vi "Fetch (Waveform To File).vi"(7 "Filename (C:\\data.txt)":path=path "C:/data.txt", 8 "error in (no error)":errorcluster, 9 "Maximum Time (200000ms)":u32=200000, 10 "Channel (0:Channel1)":u16(ring) items=["Channel1", "Channel2", "Channel3", "Channel4", "Math1", "Math2", "Math3", "Math3", "Reference1", "Reference2", "Reference3", "Reference4"], 11 "VISA resource name":refnum<visa-resource-name>) -> (0 "error out":errorcluster, 3 "VISA resource name out":refnum<visa-resource-name>)   [LabVIEW 2011, in "Tektronix 7000 Series.lvlib"]
doc: "Returns to a file the waveform that an oscilloscope acquires for a channel you specify. An acquisition that you initiate before calling this VI generates the waveform.\n\nYou first enable channels with the Configure Channel VI. Then you use the Initiate VI to start an acquisition on the enabled channels. An oscilloscope concurrently acquires waveforms for these channels and returns them in a file.\n\n<B>Note</B>: Use the Fetch Waveform To File VI only with other low-level VIs, such as the Initiate VI, the Abort VI, and the Fetch Waveform VI."
uses:
  Tektronix 7000 Series.lvlib
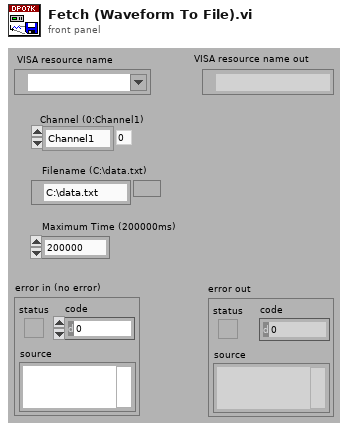
[diagram p1: front panel]
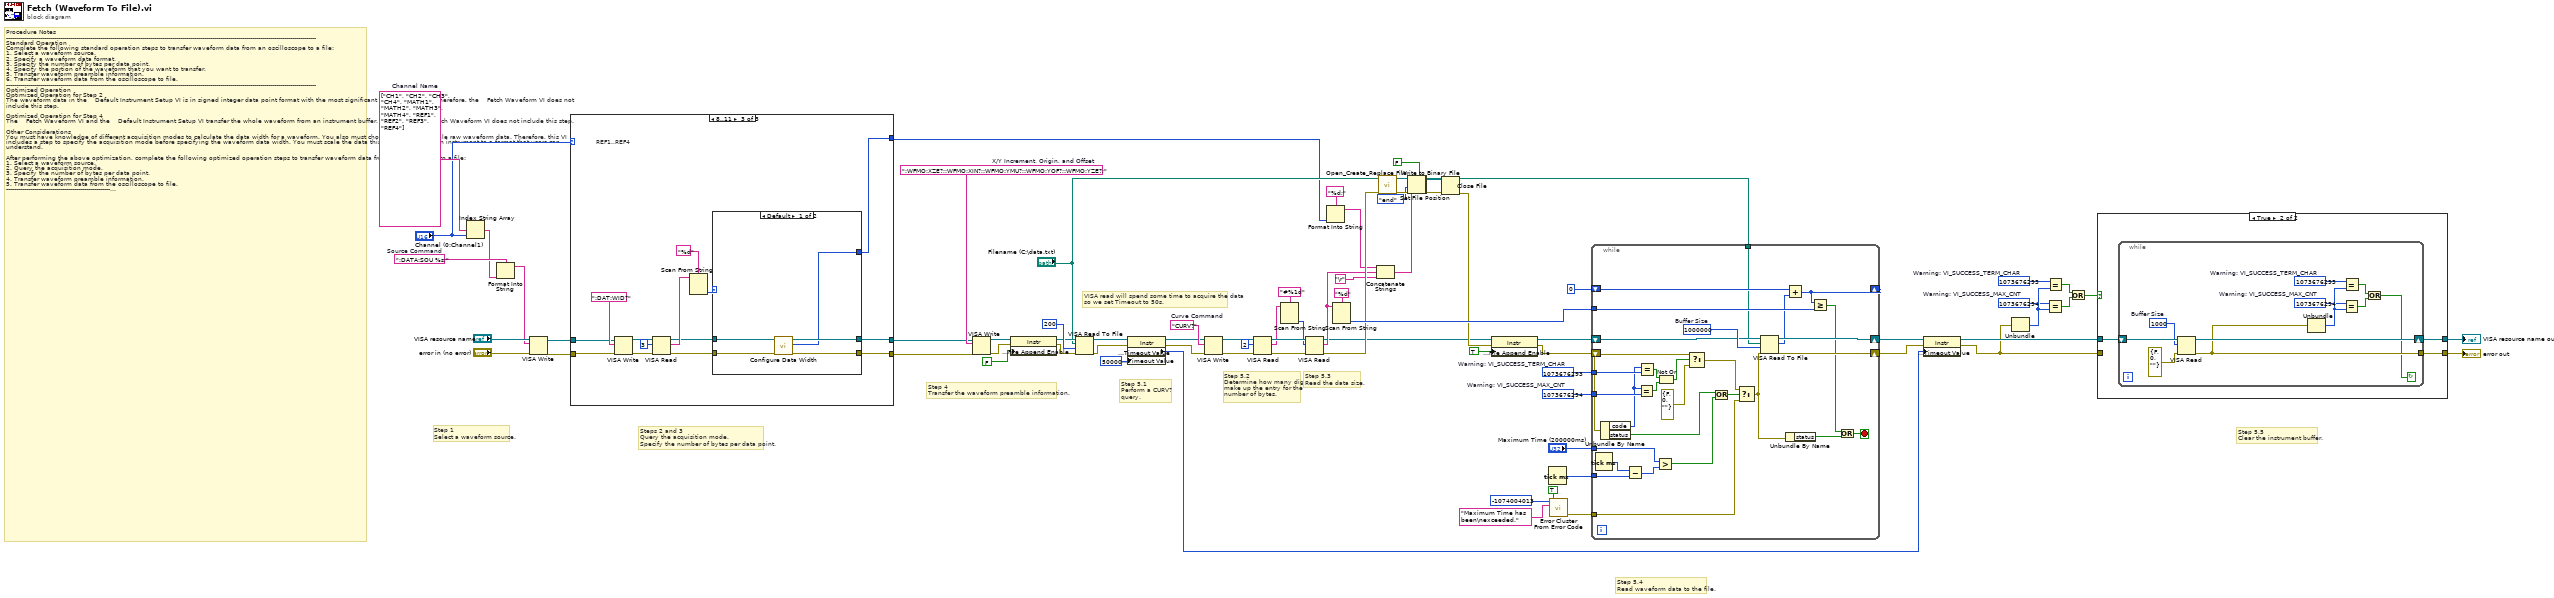
[diagram p0: block diagram]
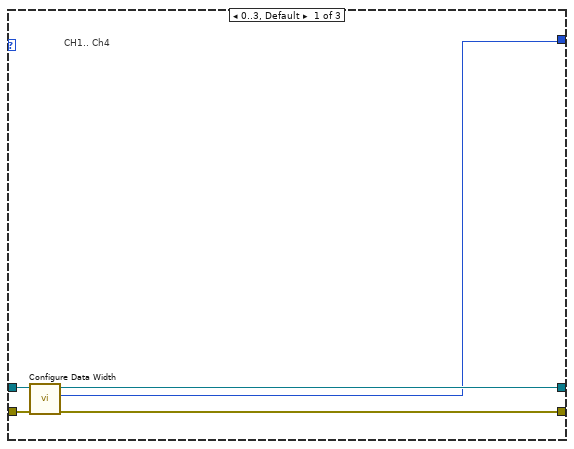
[diagram p2: hidden frame]
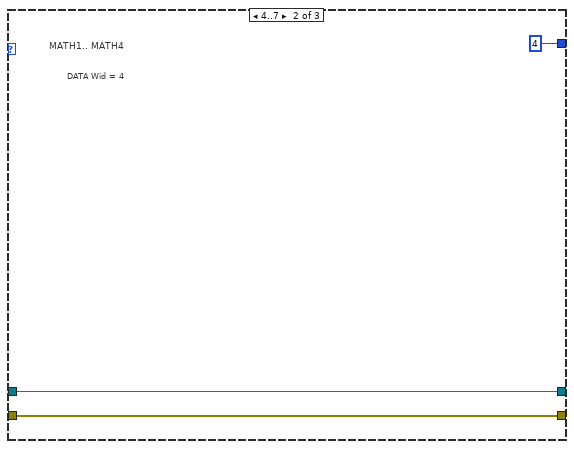
[diagram p3: hidden frame]
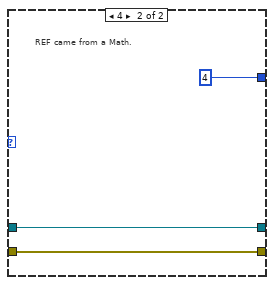
[diagram p4: hidden frame]
diagram:
  w51 = string[] ["CH1", "CH2", "CH3", "CH4", "MATH1", "MATH2", "MATH3", "MATH4", "REF1", "REF2", "REF3", "REF4"]  # Channel Name
  w57 = 1073676294  # Warning: VI_SUCCESS_MAX_CNT
  w58 = 1073676293  # Warning: VI_SUCCESS_TERM_CHAR
  w61 = 1073676294  # Warning: VI_SUCCESS_MAX_CNT
  w60 = 1073676293  # Warning: VI_SUCCESS_TERM_CHAR
  w75 = "CURV?"  # Curve Command
  w77 = ":DATA:SOU %s;"  # Source Command
  w46 = ":WFMO:XZE?;:WFMO:XIN?;:WFMO:YMU?;:WFMO:YOF?;:WFMO:YZE?;"  # X/Y Increment, Origin, and Offset
  # "VISA read will spend some time to acquire the data \nso we set Timeout to 50s."
  # "Step 4\nTransfer the waveform preamble information."
  # "Step 1\nSelect a waveform source."
  # "Steps 2 and 3\nQuery the acquisition mode. \nSpecify the number of bytes per data point."
  # "Procedure Notes\n-----------------------------------------------------------------------------------------------------------------------------------------------------------\nStandard Operation\nComplete the following standard operation steps to transfer waveform data from an oscilloscope to a file:\n1. Select a waveform source.\n2. Specify a waveform data format.\n3. Specify the number of bytes per data point.\n4. Specify the portion of the waveform that you want to transfer.\n5. Transfer waveform preamble information.\n6. Transfer waveform data from the oscilloscope to file.\n-----------------------------------------------------------------------------------------------------------------------------------------------------------\nOptimized Operation\nOptimized Operation for Step 2\nThe waveform data in the    Default Instrument Setup VI is in signed integer data point format with the most significant byte transfer first. Therefore, the    Fetch Waveform VI does not include this step.\n\nOptimized Operation for Step 4 \nThe    Fetch Waveform VI and the    Default Instrument Setup VI transfer the whole waveform from an instrument buffer. Therefore, the    Fetch Waveform VI does not include this step.\n\nOther Considerations\nYou must have knowledge of different acquisition modes to calculate the data width for a waveform. You also must choose a method to scale raw waveform data. Therefore, this VI includes a step to specify the acquisition mode before specifying the waveform data width. You must scale the data this VI retrieves from an instrument to a format that users can understand.\n\nAfter performing the above optimization, complete the following optimized operation steps to transfer waveform data from an oscilloscope to a file:\n1. Select a waveform source.\n2. Query the acquisition mode.\n3. Specify the number of bytes per data point.\n4. Transfer waveform preamble information.\n5. Transfer waveform data from the oscilloscope to file.\n-----------------------------------------------------------------------------------------------------------------------------------------------------------\nDetailed Steps\nThe following steps detail the behavior of this VI:\n1. Select a waveform source. \n2. Query and determine the acquisition mode. A correct determination is critical to steps 3 and 6.\n    -----------------------------------------------\n    Acquisition Mode |  Data Width   \n    -----------------------------------------------\n    Normal                       |   1                      \n    -----------------------------------------------\n    Peak Detect               |   1                      \n    -----------------------------------------------\n    Hi Res                        |   2                      \n    -----------------------------------------------\n    Envelope                   |   1                      \n    ----------------------------------------------- \n    Average                    |   2                      \n    -----------------------------------------------\n3. Specify the number of bytes per data point. For the Hi Res or Average acquisition modes, set the data width to 2. For all other acquisition modes, set the data width to 1.\n4. Transfer the waveform preamble information to file. Necessary preamble information includes XZero, XIncrement, YMultiplier, YOffset, and YZero. This VI uses XZero and XIncrement to configure the x-axis of output waveforms and uses YMultiplier, YOffset, and YZero to scale data values. This VI then parses the return string of the preamble query in step 6.\n5. Transfer waveform data from the oscilloscope to file.\n    5.1 Perform a CURV? query.\n    5.2 Determine how many digits make up the entry for the number of bytes.\n    5.3 Read the data size to file.\n    5.4 Call the VISA Read VI repeatedly with a buffer size of 1000000 until you obtain as much data as the data size specifies. Save the data to file.\n    5.5 Continue reading the data remaining in the instrument buffer until the buffer is empty.\n\nFile Structure:\n    XZero;XIncrement;YMultiplier;YOffset;YZero\n    Width;Date Length\n    Waveform Data"
  # "Step 5.5    \nClear the instrument buffer."
  # "Step 5.4   \nRead waveform data to the file."
  # "Step 5.3      \nRead the data size."
  # "Step 5.2      \nDetermine how many digits\nmake up the entry for the \nnumber of bytes."
  # "Step 5.1      \nPerform a CURV?\nquery."
  n1 = Index String Array(1:"Channel (0:Channel1)", 2:w51) -> (0:w76:string)  [unwired: 1 in]
  n2 = Format Into String(format string=w77, w76) -> (resulting string=w48:string)  [unwired: 2 in, 1 out]
  n3 = VISA Write(VISA resource name="VISA resource name", write buffer=w48, error in (no error)="error in (no error)") -> (VISA resource name out=w45:refnum<visa-resource-name>, error out=w44:errorcluster)  [unwired: 1 out]
  n4 = case shown="8..11" "Channel (0:Channel1)" {
    tunnel: w45 -> [w82 w85 w94]
    tunnel: w44 -> [w81 w84 w95]
    tunnel: [w80 w85 w88] -> w9
    tunnel: [w79 w84 w87] -> w8
    tunnel: [w78 u32 4 ("byte count") w86] -> w10
    frame 0..3, Default {
      # "CH1.. Ch4"
      n5 = call "Configure Data Width.vi"("error in (no error)"=w81, "VISA resource name"=w82) -> ("error out"=w79:errorcluster, "Width"=w78:i32, "VISA resource name out"=w80:refnum<visa-resource-name>)  [unwired: 7 in]
    }
    frame 4..7 {
      # "DATA Wid = 4"
      # "MATH1.. MATH4"
    }
    frame 8..11 {
      # "REF1..REF4"
      n6 = VISA Write(VISA resource name=w94, write buffer=":DAT:WID?", error in (no error)=w95) -> (VISA resource name out=w99:refnum<visa-resource-name>, error out=w98:errorcluster)  [unwired: 1 out]
      n7 = VISA Read(VISA resource name=w99, byte count=u32 3, error in (no error)=w98) -> (VISA resource name out=w90:refnum<visa-resource-name>, read buffer=w93:string, error out=w89:errorcluster)  [unwired: 1 out]
      n8 = Scan From String(format string="%d", input string=w93) -> (output 1=w91:i32)  [unwired: 3 in, 3 out]
      n9 = case shown="Default" w91 {
        tunnel: w90 -> [w104 w107]
        tunnel: w89 -> [w103 w106]
        tunnel: [w102 w107] -> w88
        tunnel: [w101 w106] -> w87
        tunnel: [w100 u32 4 ("byte count")] -> w86
        frame Default {
          n10 = call "Configure Data Width.vi"("error in (no error)"=w103, "VISA resource name"=w104) -> ("error out"=w101:errorcluster, "Width"=w100:i32, "VISA resource name out"=w102:refnum<visa-resource-name>)  [unwired: 7 in]
        }
        frame 4 {
          # "REF came from a Math."
        }
      }
    }
  }
  n11 = VISA Write(VISA resource name=w9, write buffer=w46, error in (no error)=w8) -> (VISA resource name out=w30:refnum<visa-resource-name>, error out=w27:errorcluster)  [unwired: 1 out]
  n12 = property class="Instr"(reference=w30, error in=w27, "Message Based Settings:File Append Enable"=FALSE) -> (reference out=w29:refnum<visa-resource-name>, error out=w28:errorcluster)
  n13 = VISA Read To File(8:w28, 9:u32 200 ("byte count"), 10:"Filename (C:\\data.txt)", 11:w29) -> (0:w6:errorcluster, 3:w7:refnum<visa-resource-name>)  [unwired: 1 out]
  n14 = property on="Property Node" class="Instr"(reference=w7, error in=w6, "General Settings:Timeout Value"=u32 50000) -> (reference out=w5:refnum<visa-resource-name>, error out=w4:errorcluster, "General Settings:Timeout Value"=w54:u32)
  n15 = VISA Write(VISA resource name=w5, write buffer=w75, error in (no error)=w4) -> (VISA resource name out=w43:refnum<visa-resource-name>, error out=w74:errorcluster)  [unwired: 1 out]
  n16 = VISA Read(VISA resource name=w43, byte count=u32 2, error in (no error)=w74) -> (VISA resource name out=w71:refnum<visa-resource-name>, read buffer=w69:string, error out=w70:errorcluster)  [unwired: 1 out]
  n17 = Scan From String(format string="#%1d", input string=w69) -> (output 1=w68:i32)  [unwired: 3 in, 3 out]
  n18 = VISA Read(VISA resource name=w71, byte count=w68, error in (no error)=w70) -> (VISA resource name out=w19:refnum<visa-resource-name>, read buffer=w25:string, error out=w34:errorcluster)  [unwired: 1 out]
  n19 = Format Into String(format string="%d;", w10) -> (resulting string=w21:string)  [unwired: 2 in, 1 out]
  n20 = Scan From String(format string="%d", input string=w25) -> (output 1=w35:i32)  [unwired: 3 in, 3 out]
  n21 = Concatenate Strings(w21, w25, "\r") -> (w24:string)
  n22 = call <vilib>:"Open_Create_Replace File.vi"("error in (no error)"=w34, "file path"="Filename (C:\\data.txt)") -> ("error out"=w33:errorcluster, "refnum"=w37:refnum<file>)  [unwired: 6 in, 2 out]
  n23 = Set File Position(refnum=w37, from (0:start)=enum16{"start", "end", "current"}."end" ("pos mode (0:2)"), error in=w33) -> (refnum out=w3:refnum<file>, error out=w2:errorcluster)  [unwired: 1 in]
  n24 = Write to Binary File(file (use dialog)=w3, data=w24, error in=w2, 5:FALSE ("prepend array or string size? (T)")) -> (refnum out=w36:refnum<file>, error out=w32:errorcluster)  [unwired: 2 in, 1 out]
  n25 = Close File(refnum=w36, error in=w32) -> (error out=w20:errorcluster)  [unwired: 1 out]
  n26 = property class="Instr"(reference=w19, error in=w20, "Message Based Settings:File Append Enable"=TRUE) -> (reference out=w41:refnum<visa-resource-name>, error out=w40:errorcluster)
  n27 = Tick Count (ms)() -> (millisecond timer value=w13:u32)
  n28 = call <vilib>:"Error Cluster From Error Code.vi"("show call chain? (False)"=TRUE, "error message (\"\")"="Maximum Time has been\nexceeded." ("error message (\"\")"), "error code (0)"=-1074004013) -> ("error out"=w12:errorcluster)  [unwired: 6 in]
  n29 = while {
    shift-right: [w125] -> w56
    shift-left: w41 -> [w126]
    shift-right: [w124] -> w55
    shift-left: w40 -> [w134]
    tunnel: w35 -> [w137]
    shift-right: [w122] -> _
    shift-left: 0 -> [w136]
    tunnel: w58 -> [w133]
    tunnel: w57 -> [w132]
    tunnel: "Filename (C:\\data.txt)" -> [w121]
    tunnel: "Maximum Time (200000ms)" -> [w117]
    tunnel: w13 -> [w116]
    tunnel: w12 -> [w114]
    stop <- w110 stop-if-true
    w127 = 1000000  # Buffer Size
    n30 = Tick Count (ms)() -> (millisecond timer value=w118:u32)
    n31 = Unbundle By Name(w134) -> ("code"=w131:i32, "status"=w115:bool)
    n32 = Subtract(x=w118, y=w116) -> (x-y=w119:u32)
    n33 = Equal?(x=w131, y=w132) -> (x = y?=w129:bool)
    n34 = Equal?(x=w131, y=w133) -> (x = y?=w130:bool)
    n35 = Greater?(x=w117, y=w119) -> (0:w112:bool)
    n36 = Not Or(1:w129, 2:w130) -> (0:w128:bool)
    n37 = Select(t=w134, s=w128, f=errorcluster {"status"=FALSE, "code"=0, "source"=""} ("error in (no error)")) -> (s? t:f=w113:errorcluster)
    n38 = Or(x=w115, y=w112) -> (x .or. y?=w120:bool)
    n39 = Select(t=w113, s=w120, f=w114) -> (s? t:f=w111:errorcluster)
    n40 = VISA Read To File(8:w111, 9:w127, 10:w121, 11:w126) -> (0:w124:errorcluster, 2:w123:u32, 3:w125:refnum<visa-resource-name>)
    n41 = Unbundle By Name(w111) -> ("status"=w108:bool)
    n42 = Add(x=w136, y=w123) -> (x+y=w122:u32)
    n43 = Greater Or Equal?(x=w122, y=w137) -> (x >= y?=w109:bool)
    n44 = Or(x=w109, y=w108) -> (x .or. y?=w110:bool)
  }
  n45 = property on="Property Node" class="Instr"(reference=w56, error in=w55, "General Settings:Timeout Value"=w54) -> (reference out=w53:refnum<visa-resource-name>, error out=w52:errorcluster)
  n46 = Unbundle(w52) -> ("code"=w62:i32)  [unwired: 2 out]
  n47 = Equal?(x=w61, y=w62) -> (x = y?=w64:bool)
  n48 = Equal?(x=w60, y=w62) -> (x = y?=w65:bool)
  n49 = Or(x=w65, y=w64) -> (x .or. y?=w63:bool)
  n50 = case shown="True" w63 {
    tunnel: w53 -> [w139 w142]
    tunnel: w52 -> [w138 _]
    tunnel: [w139 w141] -> w66
    tunnel: [w138 w140] -> w39
    frame False {
    }
    frame True {
      n51 = while {
        shift-right: [w152] -> w141
        shift-left: w142 -> [w153]
        tunnel: [w145] -> w140
        stop <- w144 continue-if-true
        w147 = 1073676294  # Warning: VI_SUCCESS_MAX_CNT
        w146 = 1073676293  # Warning: VI_SUCCESS_TERM_CHAR
        w151 = u32 1000  # Buffer Size
        n52 = VISA Read(VISA resource name=w153, byte count=w151, error in (no error)=errorcluster {"status"=FALSE, "code"=0, "source"=""}) -> (VISA resource name out=w152:refnum<visa-resource-name>, error out=w145:errorcluster)  [unwired: 2 out]
        n53 = Unbundle(w145) -> ("code"=w148:i32)  [unwired: 2 out]
        n54 = Equal?(x=w147, y=w148) -> (x = y?=w149:bool)
        n55 = Equal?(x=w146, y=w148) -> (x = y?=w150:bool)
        n56 = Or(x=w150, y=w149) -> (x .or. y?=w144:bool)
      }
    }
  }
  "error out" <- w39
  "VISA resource name out" <- w66
